vi "Write Self Attributes.vi"(10 "Self Attributes":refnum<data-value>, 11 "TEMPLATE Actor in":refnum<class "TEMPLATE Actor.lvclass">) -> (3 "TEMPLATE Actor out":refnum<class "TEMPLATE Actor.lvclass">)   [LabVIEW 2020, in "_Template.lvlib" / "Templates.lvlib" / "TEMPLATE jettl Actor.lvlib" / "TEMPLATE Actor.lvlib" / "TEMPLATE Actor.lvclass"]
uses:
  TEMPLATE Actor.lvclass
  TEMPLATE Actor.lvclass/TEMPLATE Actor.ctl
  jettl/jettl/Actor/Actor.lvclass
  jettl/jettl/Transport/Transport.lvclass
  jettl/jettl/Actor Attributes.ctl
  jettl/jettl/jettl.lvlib
  jettl/jettl/Msg/Msg.lvclass
  jettl/jettl/Msgs.ctl
  jettl/jettl/Msg Names.ctl
  jettl/jettl/Unified Layer.ctl
panel:
  # "This front panel should not be manipulated."
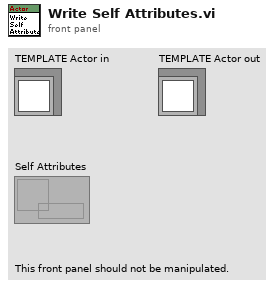
[diagram p1: front panel]
types:
  T1 = typedef "jettl.lvlib/Actor.ctl" = cluster{"Layer":T2, "Actor":refnum<class "Actor.lvclass">, "Refs":refnum<class "Refs.lvclass">}
  T2 = typedef "jettl.lvlib/Layer.ctl" = cluster{"Msgs":T3, "Msg Names":T4, "Leaf":bool, "Index":i32, "Name":string}
  T3 = typedef "jettl.lvlib/Msgs.ctl" = set{refnum<class "Msg.lvclass">}
  T4 = typedef "jettl.lvlib/Msg Names.ctl" = set{string}
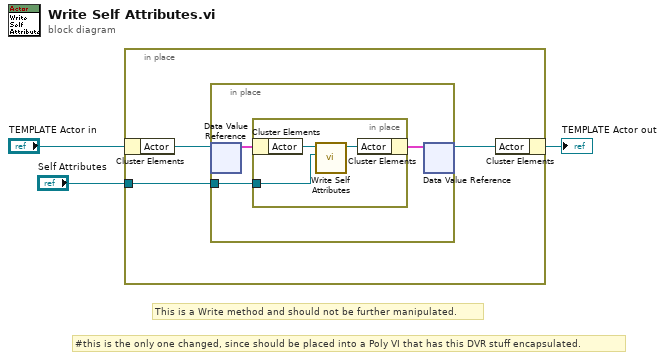
[diagram p0: block diagram]
diagram:
  # "#this is the only one changed, since should be placed into a Poly VI that has this DVR stuff encapsulated."
  # "This is a Write method and should not be further manipulated."
  n1 = in-place {
    in-place-border: "Self Attributes" -> [w6]
    n2 = in-place-cluster #1("TEMPLATE Actor in") -> ("Actor"=w5:refnum<data-value>)
    n3 = in-place {
      in-place-border: w6 -> [w7]
      n4 = in-place-dvr #2(w5) -> (w9:T1)  [unwired: 1 out]
      n5 = in-place {
        in-place-border: w7 -> [w12]
        n6 = in-place-cluster #3(w9) -> ("Actor"=w11:refnum<class "Actor.lvclass">)
        n7 = call-dynamic "Write Self Attributes.vi"("Self Attributes"=w12, "Actor in"=w11) -> ("Actor out"=w10:refnum<class "Actor.lvclass">)  [unwired: 9 in]
        n8 = in-place-cluster #3("Actor"=w10) -> (w8:T1)
      }
      n9 = in-place-dvr #2(w8) -> (w4:refnum<data-value>)  [unwired: 1 out]
    }
    n10 = in-place-cluster #1("Actor"=w4) -> (→"TEMPLATE Actor out":refnum<class "TEMPLATE Actor.lvclass">)
  }
